vi "02señalizacion 568.vi"(5 "LOGICAS":T1, 6 "ANALOGICAS":cluster{"Med OUT num":dbl, "Nombre":string}[](array[cluster]), 7 "Config Equipo":T3={"Modelo"="", "IP"="", "Puerto"=0, "Time Out"=0, "Med Princ"=0, "Time sin rx"=60, "Reintento"=60, "Ref PD 2"=200} {"Ref PD 2" max=10000 step=1; "Med Princ" items=["1", "2", "3", "4", "5", "6", "7", "8", "9", "10", "11", "12", "13", "14", "15", "16", "17", "18", "19", "20", "21", "22", "23", "24", "25", "26", "27", "28", "29", "30", "31", "32"]}) -> (2 "Error Logico":bool, 3 "Señalizacion":T2)   [LabVIEW 2010]
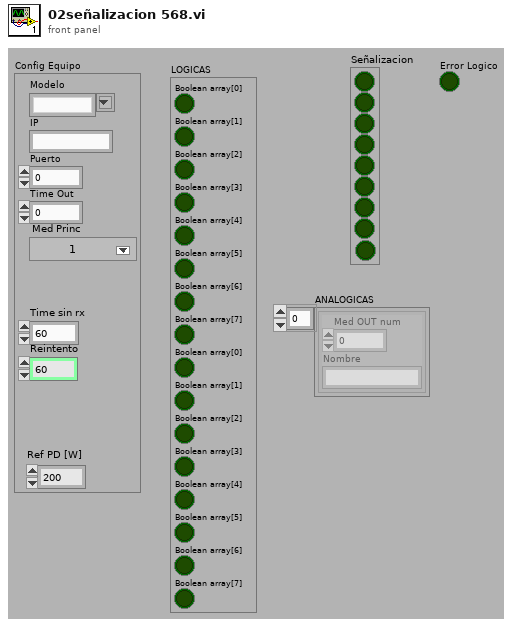
[diagram p1: front panel]
types:
  T1 = cluster{"Boolean array[0]":bool, "Boolean array[1]":bool, "Boolean array[2]":bool, "Boolean array[3]":bool, "Boolean array[4]":bool, "Boolean array[5]":bool, "Boolean array[6]":bool, "Boolean array[7]":bool, "Boolean array[0]":bool, "Boolean array[1]":bool, "Boolean array[2]":bool, "Boolean array[3]":bool, "Boolean array[4]":bool, "Boolean array[5]":bool, "Boolean array[6]":bool, "Boolean array[7]":bool}
  T2 = cluster{bool, bool, bool, bool, bool, bool, bool, bool, bool}
  T3 = cluster{"Modelo":string, "IP":string, "Puerto":u16, "Time Out":u16, "Med Princ":u16, "Time sin rx":u16, "Reintento":u16, "Ref PD 2":u16}
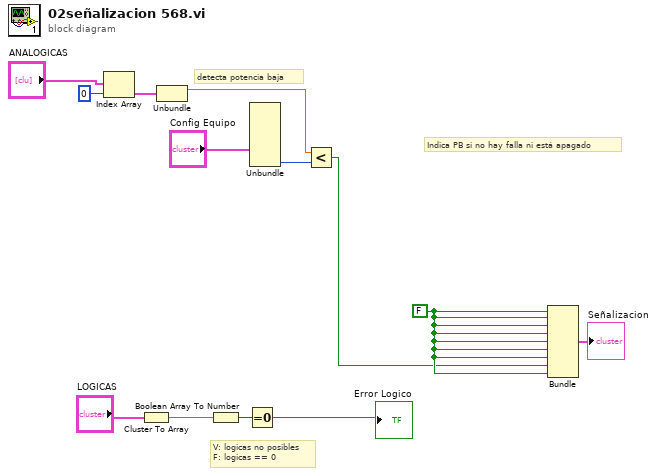
[diagram p0: block diagram]
diagram:
  w6 = FALSE
  # "V: logicas no posibles\nF: logicas == 0"
  # "Indica PB si no hay falla ni está apagado"
  # "detecta potencia baja"
  n1 = Index Array(array="ANALOGICAS", index=0 ("offset (0)")) -> (element=w9:cluster{"Med OUT num":dbl, "Nombre":string})
  n2 = Cluster To Array(cluster="LOGICAS") -> (array=w3:bool[])
  n3 = Unbundle(w9) -> ("Med OUT num"=w8:dbl)  [unwired: 1 out]
  n4 = Boolean Array To Number(Boolean array=w3) -> (number=w2:u32)
  n5 = Equal To 0?(x=w2) -> (x = 0?=→"Error Logico":bool)
  n6 = Unbundle("Config Equipo") -> ("Ref PD 2"=w13:u16)  [unwired: 7 out]
  n7 = Less?(x=w8, y=w13) -> (x < y?=w5:bool)
  n8 = Bundle(w6, w6, w6, w6, w6, w6, w6, w5, w6) -> (→"Señalizacion":T2)  [unwired: 1 out]
